vi "API Commands--Constant.vi"(8 "error in (no error)":errorcluster, 11 "VoltageUpdate in":refnum<class "VoltageUpdate.lvclass">) -> (0 "error out":errorcluster, 2 "API Commands":string[](array[string]), 3 "VoltageUpdate out":refnum<class "VoltageUpdate.lvclass">)   [LabVIEW 2016, in "VoltageUpdate.lvclass"]
uses:
  VoltageUpdate.lvclass
panel:
  # "Modify constant on block diagram"
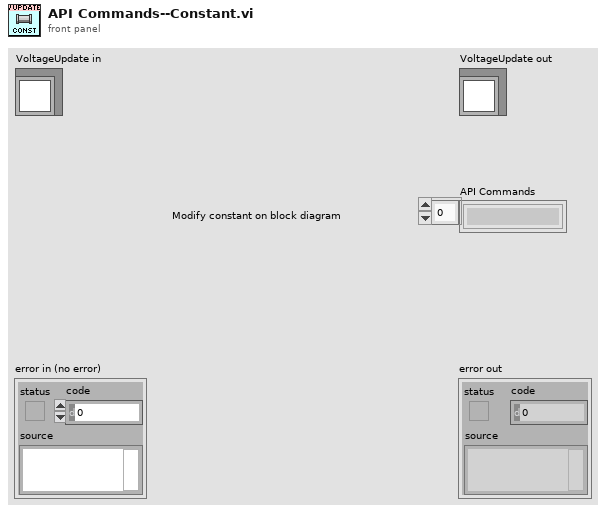
[diagram p1: front panel]
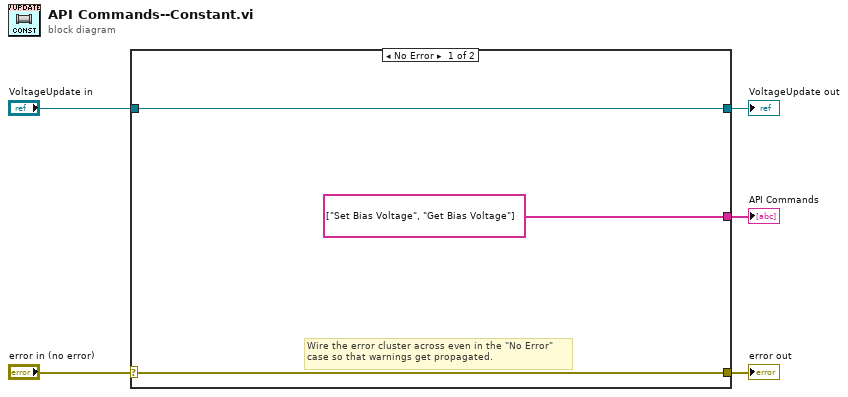
[diagram p0: block diagram]
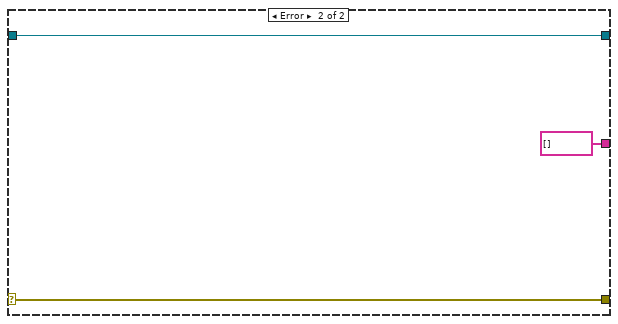
[diagram p2: hidden frame]
diagram:
  n1 = case shown="No Error" "error in (no error)" {
    selector: "error in (no error)" -> [w7 w11]
    tunnel: [w7 w11] -> w4
    tunnel: [w8 w10] -> w2
    tunnel: "VoltageUpdate in" -> [w8 w10]
    tunnel: [string[] ["Set Bias Voltage", "Get Bias Voltage"] ("Array") string[] [] ("Array")] -> w1
    frame No Error {
      # "Wire the error cluster across even in the \"No Error\"\ncase so that warnings get propagated."
    }
    frame Error {
    }
  }
  "error out" <- w4
  "VoltageUpdate out" <- w2
  "API Commands" <- w1
